vi "Temperature Grad Read.vi"   [LabVIEW 2023, in "Chiller.lvclass"]
uses:
  Chiller.lvclass
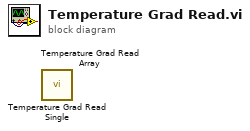
[diagram p0: block diagram]
diagram:
  n1 = call "Temperature Grad Read Single.vi"() -> ()  [unwired: 8 in, 4 out]
  n2 = call "Temperature Grad Read Array.vi"() -> ()  [unwired: 8 in, 4 out]
